vi "Reinitialize All.vi"(8 "error in (no error)":errorcluster, 10 "Initialize Edit Sensor":bool, 11 "Create Sensor View in":refnum<class "Edit Sensor View.lvclass">) -> (0 "error out":errorcluster, 3 "Create Sensor View out":refnum<class "Edit Sensor View.lvclass">)   [LabVIEW 2013, in "Edit Sensor View.lvlib" / "Edit Sensor View.lvclass"]
uses:
  Edit Sensor View.lvclass
  Edit Sensor View.lvclass/Edit Sensor View.ctl
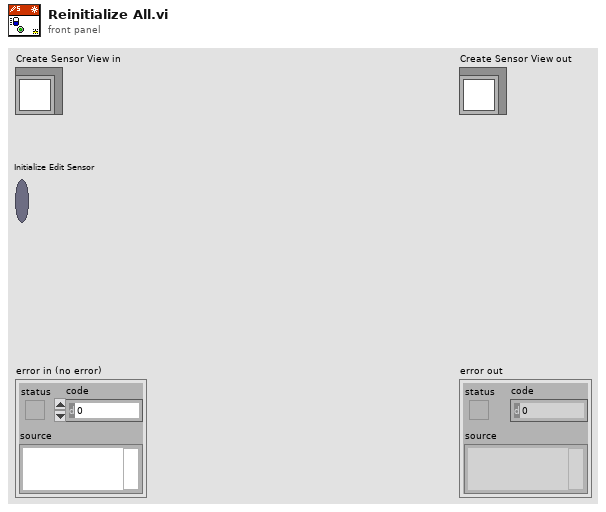
[diagram p1: front panel]
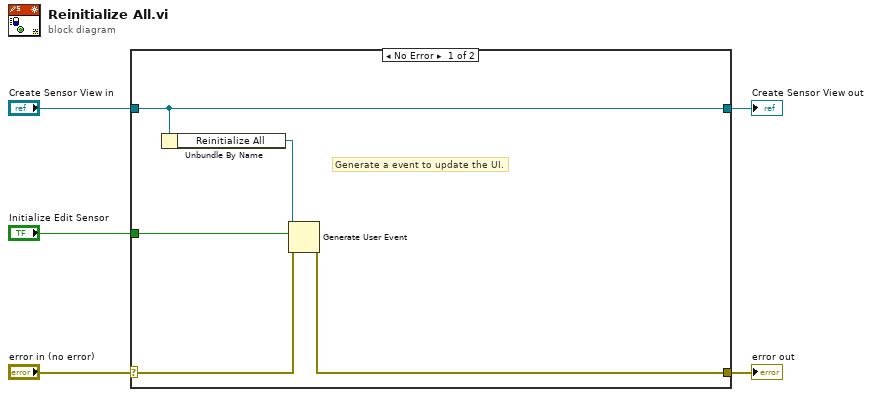
[diagram p0: block diagram]
diagram:
  n1 = case shown="No Error" "error in (no error)" {
    selector: "error in (no error)" -> [w7 w12]
    tunnel: [w6 w12] -> w4
    tunnel: [w10 w11] -> w2
    tunnel: "Create Sensor View in" -> [w10 w11]
    tunnel: "Initialize Edit Sensor" -> [w8 _]
    frame No Error {
      # "Generate a event to update the UI."
      n2 = Unbundle By Name(w10) -> ("Reinitialize All"=w9:refnum<user-event>)
      n3 = Generate User Event(user event=w9, event data cluster=w8, error in=w7) -> (error out=w6:errorcluster)  [unwired: 1 in, 1 out]
    }
    frame Error {
    }
  }
  "error out" <- w4
  "Create Sensor View out" <- w2
